vi "Get Dependency (by GUID).vi"(8 "error in (no error)":errorcluster, 10 "GUID":string, 11 "Attribute.Dependencies in":refnum<class "Attribute.Dependencies.lvclass">) -> (0 "error out":errorcluster, 1 "found":bool, 2 "Dependency":T1, 3 "Attribute.Dependencies out":refnum<class "Attribute.Dependencies.lvclass">)   [LabVIEW 2021, in "smo.lvlib" / "Attribute.Dependencies.lvclass"]
uses:
  Attribute.Dependencies.lvclass
  DependencyAttr--Cluster.ctl
  SMO/SMO.lvclass
  Attribute.Dependencies.lvclass/Attribute.Dependencies.ctl
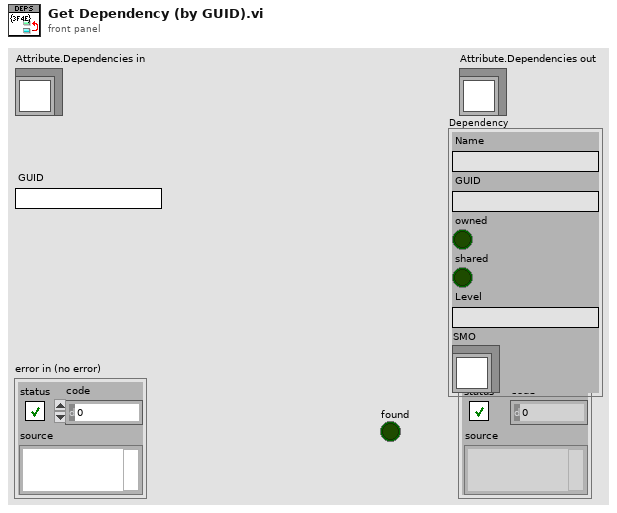
[diagram p1: front panel]
types:
  T1 = typedef "smo.lvlib/Attribute.Dependencies.lvclass/DependencyAttr--Cluster.ctl" = cluster{"Name":string, "GUID":string, "owned":bool, "shared":bool, "Level":string, "SMO":refnum<class "SMO.lvclass">}
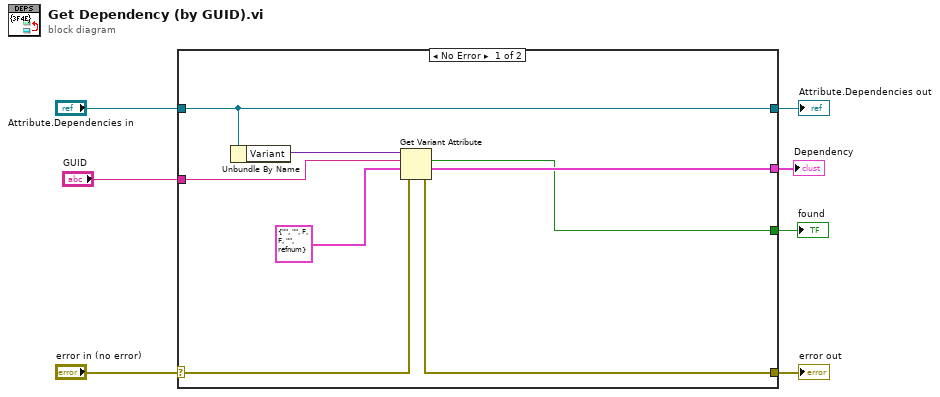
[diagram p0: block diagram]
diagram:
  n1 = case shown="No Error" "error in (no error)" {
    selector: "error in (no error)" -> [w11 w17]
    tunnel: [w10 w17] -> w6
    tunnel: [w15 w16] -> w4
    tunnel: "Attribute.Dependencies in" -> [w15 w16]
    tunnel: "GUID" -> [w13 _]
    tunnel: [w9 _] -> w2
    tunnel: [w8 _] -> w1
    frame No Error {
      n2 = Unbundle By Name(w15) -> ("Variant"=w14:variant)
      n3 = Get Variant Attribute(Variant=w14, name=w13, default value (empty Variant)=T1 {"Name"="", "GUID"="", "owned"=FALSE, "shared"=FALSE, "Level"="", "SMO"=refnum} ("Dependency"), error in=w11) -> (found=w8:bool, value=w9:T1, error out=w10:errorcluster)  [unwired: 1 out]
    }
    frame Error {
    }
  }
  "error out" <- w6
  "Attribute.Dependencies out" <- w4
  "Dependency" <- w2
  "found" <- w1
